vi "database_connection.vi"   [LabVIEW 2014]
uses:
  Program Files (x86)/National Instruments/LabVIEW 2014/vi.lib/addons/database/Connection.llb/DB Tools Open Connec (String).vi
  Program Files (x86)/National Instruments/LabVIEW 2014/vi.lib/addons/database/Connection.llb/Conn Execute.vi
  Program Files (x86)/National Instruments/LabVIEW 2014/vi.lib/addons/database/Recordset.llb/Rec Destroy - Connection.vi
  Program Files (x86)/National Instruments/LabVIEW 2014/vi.lib/addons/database/NI_Database_API.lvlib
types:
  T1 = typedef "NI_Database_API.lvlib/Conn ObjectReference.ctl" = refnum<k1>
  T2 = typedef "NI_Database_API.lvlib/Rec ObjectReference.ctl" = refnum<k1>
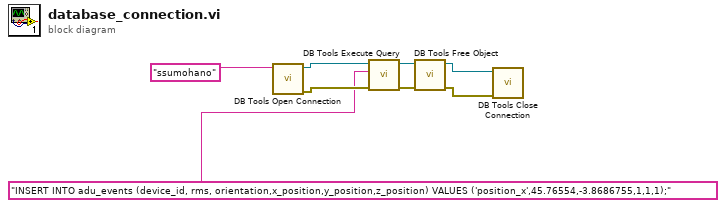
[diagram p0: block diagram]
diagram:
  n1 = call-poly "DB Tools Open Connection.vi"("connection information"="ssumohano") -> ("error out"=w6:errorcluster, "connection reference"=w7:T1)  [unwired: 7 in]
  n2 = call-poly "DB Tools Execute Query.vi"("error in (no error)"=w6, "SQL query"="INSERT INTO adu_events (device_id, rms, orientation,x_position,y_position,z_position) VALUES ('position_x',45.76554,-3.8686755,1,1,1);", "connection reference"=w7) -> ("error out"=w4:errorcluster, "recordset reference"=w3:T2)  [unwired: 5 in]
  n3 = call-poly "DB Tools Free Object.vi"("error in (no error)"=w4, "recordset reference"=w3) -> ("error out"=w2:errorcluster, "connection reference"=w1:T1)  [unwired: 8 in]
  n4 = call "DB Tools Close Connection.vi"("error in (no error)"=w2, "connection reference"=w1) -> ()  [unwired: 5 in, 1 out]
